vi "coil exclusion times.vi"(9 "buffer (s) after":dbl=0.05 format="%#_13g", 10 "buffer (s) before":dbl=0.02 format="%#_13g", 11 "coil elements":T1[](array[typedef])) -> (3 "coil exclusion times":cluster{dbl, dbl}[](array[cluster]))   [LabVIEW 2017]
uses:
  typedefs/reading.ctl
  typedefs/readingType.ctl
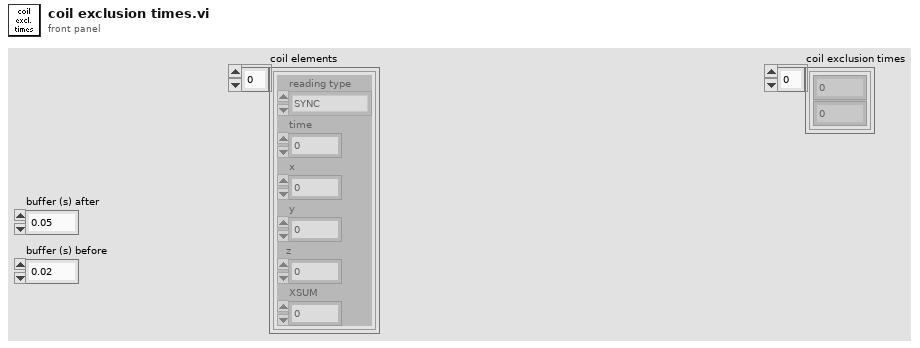
[diagram p1: front panel]
types:
  T1 = typedef "reading.ctl" = cluster{"reading type":T2, "time":fxp<+,48,48>, "x":sgl, "y":sgl, "z":sgl, "XSUM":u8}
  T2 = typedef "readingType.ctl" = enum8{"SYNC", "DETVAL", "COILI", "MAGVEC", "ACCVEC", "CROSSING", "MAGVEC0", "MAGVEC1", "MAGVEC2", "MAGVEC3", "MAGVEC4", "MAGVEC5", "MAGVEC6", "MAGVEC7"}
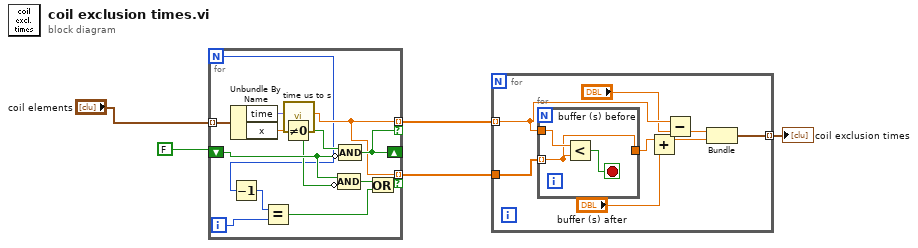
[diagram p0: block diagram]
diagram:
  n1 = for {
    N -> [w8]
    tunnel: "coil elements" -> [w17] mode=indexing
    tunnel: [w12] -> w4 mode=indexing if=w15
    shift-right: [w15] -> _
    shift-left: FALSE -> [w14]
    tunnel: [w12] -> w3 mode=indexing if=w10
    i -> [w9]
    n2 = Unbundle By Name(w17) -> ("time"=w16:fxp<+,48,48>, "x"=w18:sgl)
    n3 = Decrement(x=w8) -> (x-1=w7:i32)
    n4 = Equal?(x=w7, y=w9) -> (x = y?=w6:bool)
    n5 = Not Equal To 0?(x=w18) -> (x != 0?=w13:bool)
    n6 = call "time us to s.vi"("time (us)"=w16) -> ("time (s)"=w12:dbl)  [unwired: 10 in]
    n7 = Compound Arithmetic op=AND(w14, invert w13) -> (w11:bool)
    n8 = Compound Arithmetic op=AND(w13, invert w14) -> (w15:bool)
    n9 = Or(x=w11, y=w6) -> (x .or. y?=w10:bool)
  }
  n10 = for {
    tunnel: w4 -> [w24] mode=indexing
    tunnel: w3 -> [w26]
    tunnel: [w19] -> w1 mode=indexing
    n11 = for {
      tunnel: w24 -> [w29]
      tunnel: w26 -> [w27] mode=indexing
      tunnel: [w27] -> w25
      stop <- w28 stop-if-true
      n12 = Less?(x=w29, y=w27) -> (x < y?=w28:bool)
    }
    n13 = Add(x=w25, y="buffer (s) after") -> (x+y=w21:dbl)
    n14 = Subtract(x=w24, y="buffer (s) before") -> (x-y=w23:dbl)
    n15 = Bundle(w23, w21) -> (w19:cluster{dbl, dbl})  [unwired: 1 in]
  }
  "coil exclusion times" <- w1
